vi "WPI_DashboardRetrieveStatusInfo.vi"(9 "Window Mode Notifier":refnum<notifier>, 11 "TCP Cnx":refnum<k5>) -> (0 "Power and Errors":T2, 1 "Robot Metrics":T3, 2 "Status Info":T5, 3 "Control Info":T4 {"Team Station" items=["Red 1", "Red 2", "Red 3", "Blue 1", "Blue 2", "Blue 3"]}, 4 "Robot Mode":T1(ring), 5 "Process?":bool)   [LabVIEW 2025]
uses:
  <vilib>/Rock Robotics/WPI/Dashboard/WPI_DashboardLogging Global.vi
panel:
  # "CAN Metrics\nJS HID Outputs\nFree Mem"
  # "Need to merge in TCP info too"
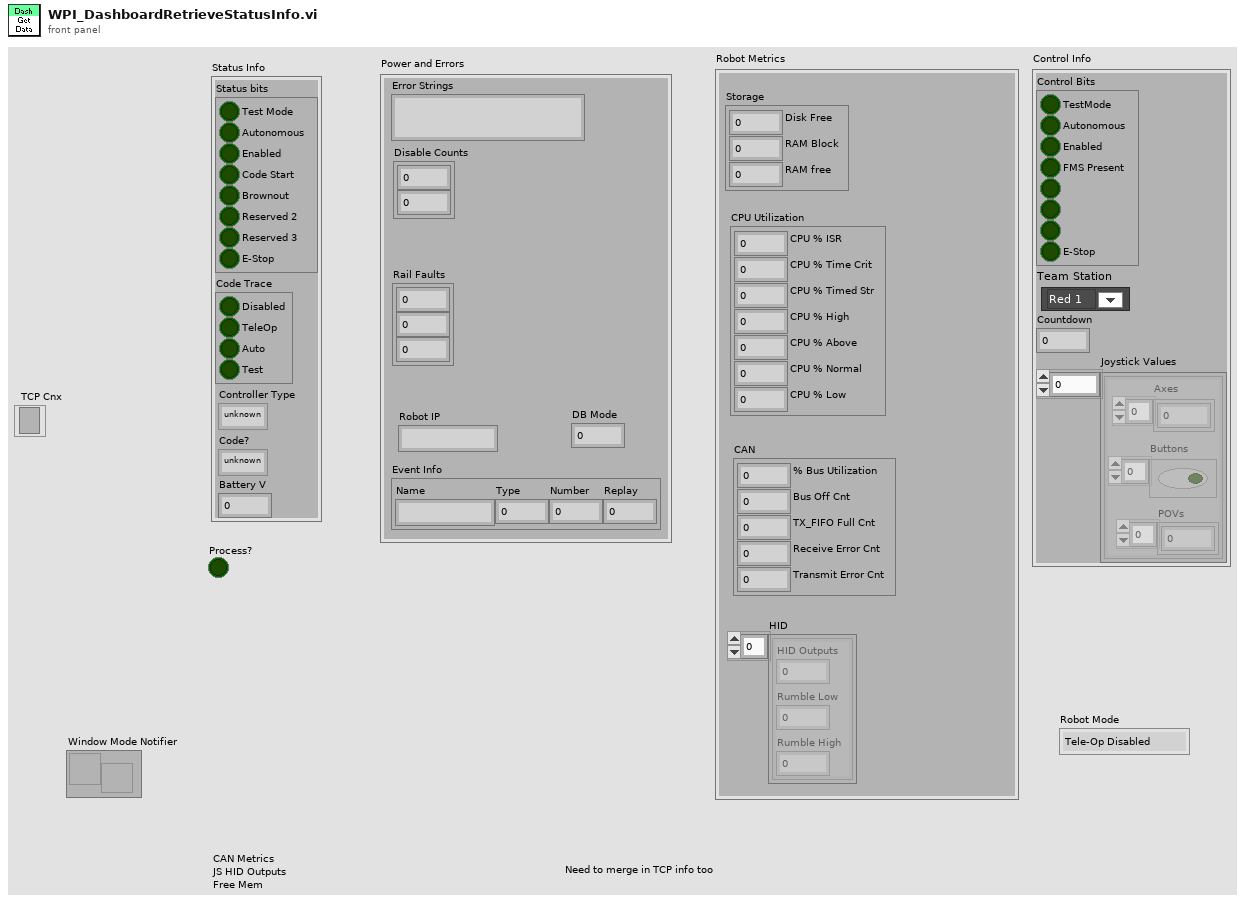
[diagram p1: front panel]
types:
  T1 = enum8{"Tele-Op Disabled", "Tele-Op Enabled", "Auto Disabled", "Auto Enabled", "Test Disabled", "Test Enabled", "Disconnected", "No Code", "E-Stop"}
  T2 = cluster{"Error Strings":string, "Disable Counts":cluster{u16, u16}, "Rail Faults":cluster{u16, u16, u16}, "Robot IP":string, "DB Mode":u8, "Event Info":cluster{"Name":string, "Type":u8, "Number":u16, "Replay":u8}}
  T3 = cluster{"Storage":cluster{"Disk Free":u64, "RAM Block":u32, "RAM free":u32}, "CPU Utilization":cluster{"CPU % ISR":sgl, "CPU % Time Crit":sgl, "CPU % Timed Str":sgl, "CPU % High":sgl, "CPU % Above":sgl, "CPU % Normal":sgl, "CPU % Low":sgl}, "CAN":cluster{"% Bus Utilization":sgl, "Bus Off Cnt":u32, "TX_FIFO Full Cnt":u32, "Receive Error Cnt":u8, "Transmit Error Cnt":u8}, "HID":cluster{"HID Outputs":u32, "Rumble Low":u16, "Rumble High":u16}[]}
  T4 = cluster{"Control Bits":cluster{"TestMode":bool, "Autonomous":bool, "Enabled":bool, "FMS Present":bool, bool, bool, bool, "E-Stop":bool}, "Team Station ":u8, "Countdown":sgl, "Joystick Values":cluster{"Axes":dbl[], "Buttons":bool[], "POVs":i16[]}[]}
  T5 = cluster{"Status bits":cluster{"Test Mode":bool, "Autonomous":bool, "Enabled":bool, "Code Start":bool, "Brownout":bool, "Reserved 2":bool, "Reserved 3":bool, "E-Stop":bool}, "Code Trace":cluster{"Disabled":bool, "TeleOp":bool, "Auto":bool, "Test":bool}, "Controller Type":enum16{"unknown", "cRIO", "roboRio"}, "Code?":enum16{"unknown", "noCode", "code"}, "Battery V":dbl}
  T6 = cluster{"TestMode":bool, "Autonomous":bool, "Enabled":bool, "FMS Present":bool, bool, bool, bool, "E-Stop":bool}
  T7 = enum16{"Standard", "Buffered", "CRLF", "Immediate"}
  T8 = cluster{"UDP Status":string, "TCP":string, "UDP Control":string}
  T9 = cluster{"Error Strings":string, "Disable Counts":cluster{u16, u16}, "Rail Faults":cluster{u16, u16, u16}, "Robot IP":string, "Mode":u8, "Event Info":cluster{"Name":string, "Type":u8, "Number":u16, "Replay":u8}}
  T10 = cluster{"Boolean array":cluster{"Boolean array[0]":bool, "Boolean array[1]":bool, "Boolean array[2]":bool, "Boolean array[3]":bool, "Boolean array[4]":bool, "Boolean array[5]":bool, "Boolean array[6]":bool, "Boolean array[7]":bool}, u8, "Countdown":sgl, cluster{dbl[], bool[], i16[]}[]}
  T11 = cluster{cluster{"Disk Free":u64, "RAM Block":u32, "RAM free":u32}, cluster{"CPU Load ISR":sgl, "CPU Load Time Critical Pr":sgl, "CPU Load Timed Str Pr":sgl, "CPU Load High Pr":sgl, "CPU Load Above Normal Pr":sgl, "CPU Load Normal Pr":sgl, "CPU Load Low Pr":sgl}, cluster{"% Bus Utilization":sgl, "Bus Off Cnt":u32, "TX_FIFO Full Cnt":u32, "Receive Error Cnt":u8, "Transmit Error Cnt":u8}, cluster{"HID Outputs":u32, "Rumble Low":u16, "Rumble High":u16}[]}
  T12 = cluster{"Status":cluster{"Test Mode":bool, "Autonomous":bool, "Enabled":bool, "Code Start":bool, "Brownout":bool, "Reserved 2":bool, "Reserved 3":bool, "E-Stop":bool}, cluster{bool, bool, bool, bool}, "ctrl":enum16{"unknown", "cRIO", "roboRio"}, "code?":enum16{"unknown", "noCode", "code"}, dbl}
  T13 = cluster{"Boolean array[0]":bool, "Boolean array[1]":bool, "Boolean array[2]":bool, "Boolean array[3]":bool, "Boolean array[4]":bool, "Boolean array[5]":bool, "Boolean array[6]":bool, "Boolean array[7]":bool}
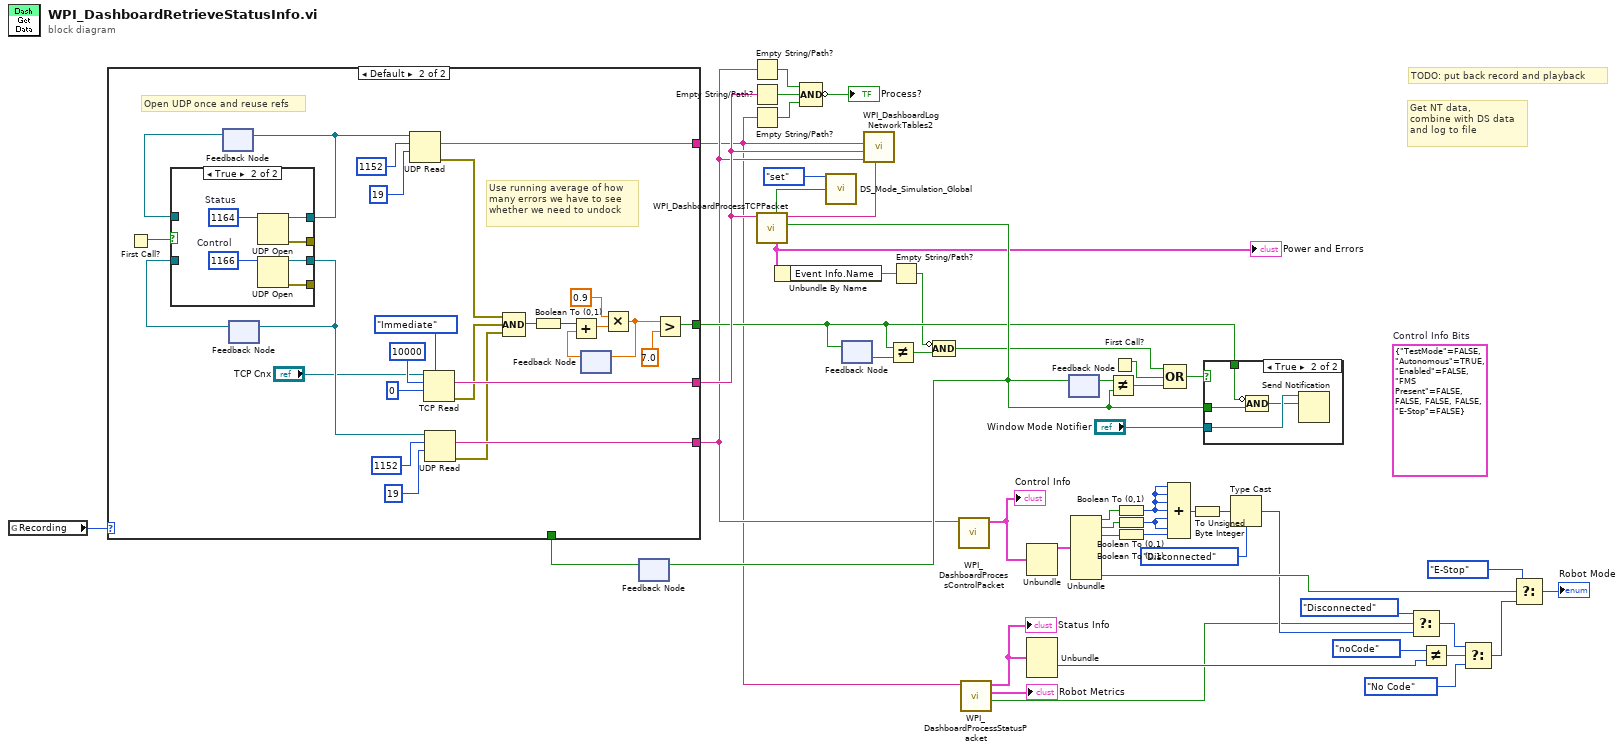
[diagram p0: block diagram]
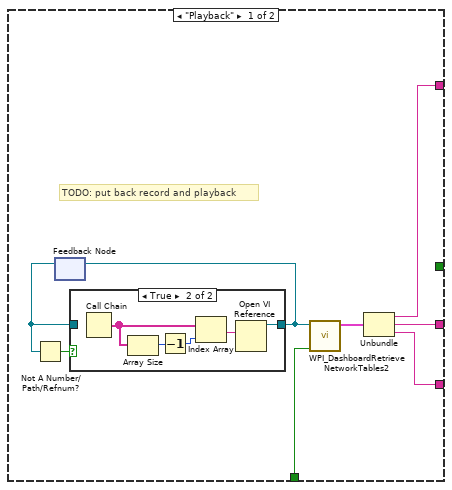
[diagram p2: hidden frame]
diagram:
  (unwired) T6 {"TestMode"=FALSE, "Autonomous"=TRUE, "Enabled"=FALSE, "FMS Present"=FALSE, FALSE, FALSE, FALSE, "E-Stop"=FALSE}  # Control Info Bits
  # "Get NT data,\ncombine with DS data\nand log to file"
  # "TODO: put back record and playback"
  n1 = global read "WPI_DashboardLogging Global.vi" "Recording"() -> (w16:enum32{"Stop", "Record", "Playback"})
  n2 = feedback #1() -> (w17:bool)  [unwired: 1 in]
  n3 = case shown="Default" w16 {
    tunnel: [w56 w84] -> w7
    tunnel: [w57 w83] -> w6
    tunnel: [w55 w82] -> w19
    tunnel: w17 -> [w54 _]
    tunnel: [_ w65] -> w15
    frame "Playback" {
      # "TODO: put back record and playback"
      n4 = feedback #2() -> (w53:refnum<vi>)  [unwired: 1 in]
      n5 = Not A Number/Path/Refnum?(number/path/refnum=w53) -> (NaN/Path/Refnum?=w52:bool)
      n6 = case shown="True" w52 {
        tunnel: w53 -> [w59 _]
        tunnel: [w59 w63] -> w51
        frame False {
        }
        frame True {
          n7 = Call Chain() -> (call chain=w62:string[])
          n8 = Array Size(array=w62) -> (size(s)=w61:i32)
          n9 = Decrement(x=w61) -> (x-1=w60:i32)
          n10 = Index Array(array=w62, index=w60) -> (element=w64:string)
          n11 = Open VI Reference(vi path=w64) -> (vi reference=w63:refnum<vi>)  [unwired: 5 in, 1 out]
        }
      }
      n12 = feedback-in #2(w51) -> ()
      n13 = call <vilib>:"WPI_DashboardRetrieve NetworkTables2.vi"("Docked Window"=w54, "DB Main Ref"=w51) -> ("Strings"=w58:T8)  [unwired: 9 in]
      n14 = Unbundle(w58) -> ("UDP Status"=w57:string, "TCP"=w55:string, "UDP Control"=w56:string)
    }
    frame Default {
      # "Use running average of how\nmany errors we have to see\nwhether we need to undock"
      # "Open UDP once and reuse refs"
      n15 = First Call?() -> (First Call?: T/F=w81:bool)
      n16 = feedback #3() -> (w79:refnum<k16>)  [unwired: 1 in]
      n17 = feedback #4() -> (w77:refnum<k16>)  [unwired: 1 in]
      n18 = case shown="True" w81 {
        tunnel: [w93 w97] -> w80
        tunnel: [_ w96] -> _
        tunnel: [w92 w95] -> w78
        tunnel: [_ w94] -> _
        tunnel: w79 -> [w93 _]
        tunnel: w77 -> [w92 _]
        frame False {
        }
        frame True {
          w98 = u16 1166  # Control
          w99 = u16 1164  # Status
          n19 = UDP Open(11:w99) -> (port=w97:refnum<k16>, 0:w96:errorcluster)  [unwired: 2 in, 3 out]
          n20 = UDP Open(11:w98) -> (port=w95:refnum<k16>, 0:w94:errorcluster)  [unwired: 2 in, 3 out]
        }
      }
      n21 = feedback-in #3(w80) -> ()
      n22 = feedback-in #4(w78) -> ()
      n23 = UDP Read(connection ID=w80, max size (548)=1152, timeout ms (25000)=19 ("length (rest)")) -> (data out=w83:string, error out=w75:errorcluster)  [unwired: 1 in, 3 out]
      n24 = TCP Read(connection ID="TCP Cnx", bytes to read=10000 ("timeout ms (25000)"), 7:T7."Immediate" ("mode (standard)"), 9:0 ("timeout ms (25000)")) -> (data out=w82:string, error out=w74:errorcluster)  [unwired: 1 in, 1 out]
      n25 = UDP Read(connection ID=w78, max size (548)=1152, timeout ms (25000)=19 ("length (rest)")) -> (data out=w84:string, error out=w73:errorcluster)  [unwired: 1 in, 3 out]
      n26 = Compound Arithmetic op=AND(w75, w74, w73) -> (w72:bool)
      n27 = Boolean To (0,1)(Boolean=w72) -> (0, 1=w71:i16)
      n28 = feedback #5() -> (w70:dbl)  [unwired: 1 in]
      n29 = Add(x=w71, y=w70) -> (x+y=w69:dbl)
      n30 = Multiply(x=0.9 ("timeout ms (25000)"), y=w69) -> (x*y=w67:dbl)
      n31 = feedback-in #5(w67) -> ()
      n32 = Greater?(x=w67, y=7.0 ("timeout ms (25000)")) -> (0:w65:bool)
    }
  }
  n33 = Empty String/Path?(string/path=w7) -> (empty?=w13:bool)
  n34 = Empty String/Path?(string/path=w19) -> (empty?=w12:bool)
  n35 = Empty String/Path?(string/path=w6) -> (empty?=w11:bool)
  n36 = call <vilib>:"WPI_DashboardProcessTCPPacket.vi"("data in"=w19) -> ("Docked"=w18:bool, "Robot IP"=w8:string, "Power and Errors"=w5:T9, "Simulated"=w20:bool)  [unwired: 6 in, 1 out]
  "Power and Errors" <- w5
  n37 = feedback-in #1(w18) -> ()
  n38 = Unbundle By Name(w5) -> ("Event Info.Name"=w4:string)
  n39 = Compound Arithmetic op=AND(w13, w12, w11) -> (invert →"Process?":bool)
  n40 = call <vilib>:"DS_Mode_Simulation_Global.vi"("menu"=enum16{"set", "get"}."set", "simulated? in"=w20) -> ()  [unwired: 12 in, 2 out]
  n41 = feedback #6() -> (w14:bool)  [unwired: 1 in]
  n42 = feedback-in #6(w15) -> ()
  n43 = call <vilib>:"WPI_DashboardLog NetworkTables2.vi"("Robot IP"=w8, "UDP Control"=w7, "TCP"=w19, "UDP Status"=w6) -> ()  [unwired: 8 in]
  n44 = Not Equal?(x=w15, y=w14) -> (x != y?=w2:bool)
  n45 = Empty String/Path?(string/path=w4) -> (empty?=w3:bool)
  n46 = Compound Arithmetic op=AND(invert w3, w2) -> (w1:bool)
  n47 = call <vilib>:"WPI_DashboardProcessControlPacket.vi"("data in"=w7) -> ("Control Info"=w42:T10)  [unwired: 10 in]
  "Control Info" <- w42
  n48 = call <vilib>:"WPI_DashboardProcessStatusPacket.vi"("data in"=w6) -> ("Disconnected"=w22:bool, "Robot Metrics"=→"Robot Metrics":T11, "Status Cluster"=w34:T12)  [unwired: 8 in]
  "Status Info" <- w34
  n49 = Unbundle(w42) -> ("Boolean array"=w41:T13)  [unwired: 3 out]
  n50 = Unbundle(w34) -> ("code?"=w30:enum16{"unknown", "noCode", "code"})  [unwired: 4 out]
  n51 = feedback #7() -> (w45:bool)  [unwired: 1 in]
  n52 = feedback-in #7(w18) -> ()
  n53 = Unbundle(w41) -> ("Boolean array[0]"=w36:bool, "Boolean array[1]"=w37:bool, "Boolean array[2]"=w39:bool, "Boolean array[7]"=w33:bool)  [unwired: 4 out]
  n54 = Not Equal?(x=w45, y=w18) -> (x != y?=w46:bool)
  n55 = First Call?() -> (First Call?: T/F=w47:bool)
  n56 = Boolean To (0,1)(Boolean=w36) -> (0, 1=w35:i16)
  n57 = Boolean To (0,1)(Boolean=w37) -> (0, 1=w38:i16)
  n58 = Boolean To (0,1)(Boolean=w39) -> (0, 1=w40:i16)
  n59 = Compound Arithmetic op=OR(w1, w47, w46) -> (w48:bool)
  n60 = Compound Arithmetic op=ADD(w35, w35, w35, w35, w38, w38, w40) -> (w26:i16)
  n61 = To Unsigned Byte Integer(number=w26) -> (unsigned 8bit integer=w21:u8)
  n62 = case shown="True" w48 {
    tunnel: "Window Mode Notifier" -> [_ w103]
    tunnel: w18 -> [_ w101]
    tunnel: w15 -> [_ w102]
    frame False {
    }
    frame True {
      n63 = Compound Arithmetic op=AND(invert w102, w101) -> (w100:bool)
      n64 = Send Notification(notification=w100, notifier=w103) -> ()  [unwired: 1 in, 2 out]
    }
  }
  n65 = Type Cast(type=T1."Disconnected" ("Mode"), x=w21) -> (*(type *) &x=w25:T1)
  n66 = Select(t=T1."Disconnected" ("Mode"), s=w22, f=w25) -> (s? t:f=w10:T1)
  n67 = Not Equal?(x=enum16{"unknown", "noCode", "code"}."noCode" ("code?"), y=w30) -> (x != y?=w29:bool)
  n68 = Select(t=w10, s=w29, f=T1."No Code" ("Mode")) -> (s? t:f=w28:T1)
  n69 = Select(t=T1."E-Stop" ("Mode"), s=w33, f=w28) -> (s? t:f=→"Robot Mode":T1)
